vi "uTransport_Event_SendMsg.vi"(8 "error in (no error)":errorcluster, 10 "Msg":refnum<class "uMsg.lvclass">, 11 "uTransport_Event in":refnum<class "uTransport_Event.lvclass">) -> (0 "error out":errorcluster, 3 "uTransport_Event out":refnum<class "uTransport_Event.lvclass">)   [LabVIEW 2021, in "uFramework.lvlib" / "uTransport_Event.lvclass"]
uses:
  uTransport_Event.lvclass
  uMsg/uMsg.lvclass
  uTransport_Event.lvclass/uTransport_Event.ctl
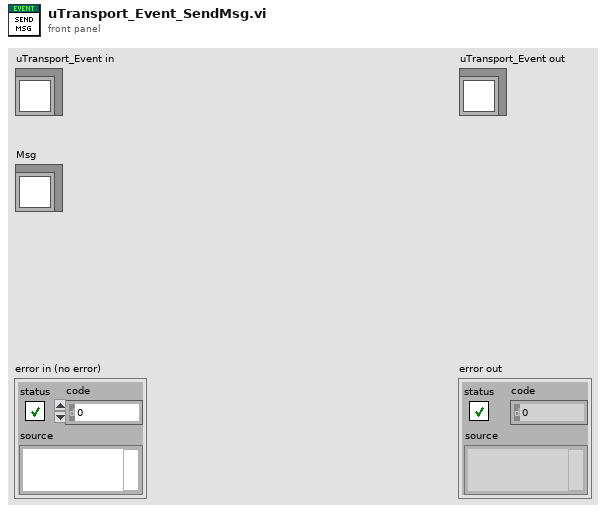
[diagram p1: front panel]
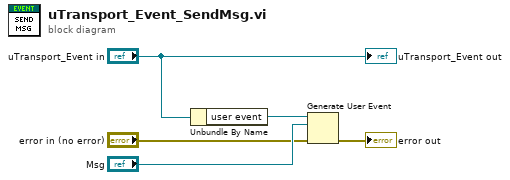
[diagram p0: block diagram]
diagram:
  n1 = Unbundle By Name("uTransport_Event in") -> ("user event"=w5:refnum<user-event>)
  n2 = Generate User Event(user event=w5, event data cluster="Msg", error in="error in (no error)") -> (error out=→"error out":errorcluster)  [unwired: 1 in, 1 out]
  "uTransport_Event out" <- "uTransport_Event in"
